vi "Piston Toggle.vi"(1 "Input":bool, 2 "Invert?":bool) -> (0 "Output":T1)   [LabVIEW 2019]
uses:
  <vilib>/Rock Robotics/WPI/Solenoid/WPI_SolenoidValue.ctl
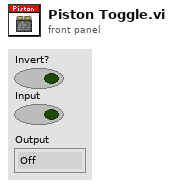
[diagram p1: front panel]
types:
  T1 = typedef "WPI_SolenoidValue.ctl" = enum16{"Off", "On", "Forward", "Reverse"}
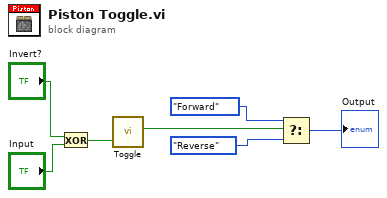
[diagram p0: block diagram]
diagram:
  n1 = Exclusive Or(1:"Input", 2:"Invert?") -> (0:w2:bool)
  n2 = call "Toggle.vi"("Input"=w2) -> ("Output"=w1:bool)  [unwired: 10 in]
  n3 = Select(t=WPI_SolenoidValue."Forward" ("Value"), s=w1, f=WPI_SolenoidValue."Reverse" ("Value")) -> (s? t:f=→"Output":T1)
